vi "Compute Distance.vi"(6 "Camera Info":T1, 8 "Height from ground of target":dbl, 10 "Bounding Box":T2) -> (2 "Bounding Box (Rad)":T2, 3 "Distance Info":cluster{dbl, dbl, dbl})   [LabVIEW 2012]
doc: "Using the camera lens information and the real world width of the target, determine the distance to the target."
uses:
  CameraResolutionInfo.ctl
panel:
  in  "Target delta-height":dbl
  # "ORIGINAL\n48\n43.5"
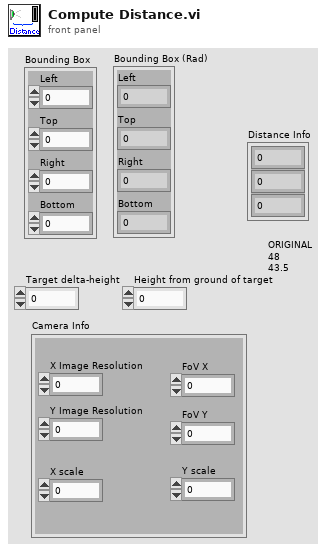
[diagram p1: front panel]
types:
  T1 = typedef "CameraResolutionInfo.ctl" = cluster{"X Image Resolution":i32, "Y Image Resolution":i32, "FoV X":dbl, "FoV Y":dbl, "X scale":dbl, "Y scale":dbl}
  T2 = cluster{"Left":dbl, "Top":dbl, "Right":dbl, "Bottom":dbl}
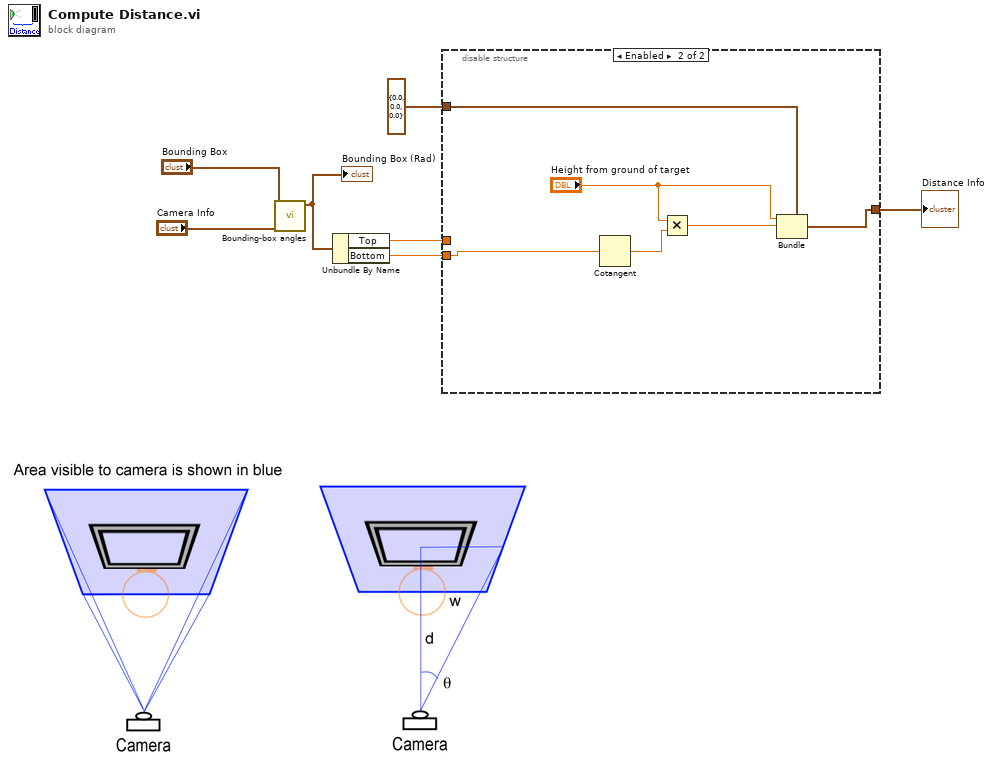
[diagram p0: block diagram]
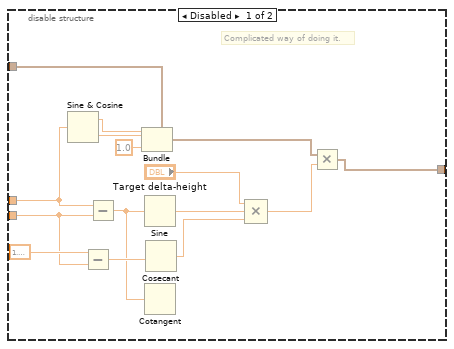
[diagram p2: hidden frame]
diagram:
  n1 = call "Bounding-box angles.vi"("Camera Info"="Camera Info", "Bounding Box"="Bounding Box") -> ("Bounding box (radians)"=w5:T2)  [unwired: 9 in]
  "Bounding Box (Rad)" <- w5
  n2 = Unbundle By Name(w5) -> ("Top"=w1:dbl, "Bottom"=w4:dbl)
  n3 = disable-structure shown="Enabled" {
    disable-tunnel: w4 -> [w21 w28]
    disable-tunnel: [w10 w24] -> w3
    disable-tunnel: cluster{dbl, dbl, dbl} {0.0, 0.0, 0.0} -> [w9 w27]
    disable-tunnel: w1 -> [w8 _]
    frame Disabled {
      # "Complicated way of doing it."
      n4 = Sine & Cosine(0:w8) -> (1:w15:dbl, 2:w14:dbl)
      n5 = Subtract(x=1.5707963267948966, y=w21) -> (x-y=w20:dbl)
      n6 = Subtract(x=w8, y=w21) -> (x-y=w11:dbl)
      n7 = Bundle(cluster=w9, w15, w14, 1.0) -> (w19:cluster{dbl, dbl, dbl})
      n8 = Sine(x=w11) -> (sin(x)=w17:dbl)
      n9 = Cotangent(1:w11) -> ()  [unwired: 1 out]
      n10 = Cosecant(1:w20) -> (0:w18:dbl)
      n11 = Compound Arithmetic op=MULTIPLY("Target delta-height", w17, w18) -> (w13:dbl)
      n12 = Multiply(x=w19, y=w13) -> (x*y=w10:cluster{dbl, dbl, dbl})
    }
    frame Enabled {
      n13 = Cotangent(1:w28) -> (0:w26:dbl)
      n14 = Multiply(x="Height from ground of target", y=w26) -> (x*y=w25:dbl)
      n15 = Bundle(cluster=w27, "Height from ground of target", w25) -> (w24:cluster{dbl, dbl, dbl})  [unwired: 1 in]
    }
  }
  "Distance Info" <- w3
